vi "Read File interpreter.lvclass.vi"(8 "error in (no error)":errorcluster, 11 "AutoExp in":refnum<class "AutoExp.lvclass">) -> (0 "error out":errorcluster, 2 "File interpreter.lvclass":refnum<class "File interpreter.lvclass">, 3 "AutoExp out":refnum<class "AutoExp.lvclass">)   [LabVIEW 2018]
uses:
  AutoExp.lvclass
  File interpreter/File interpreter.lvclass
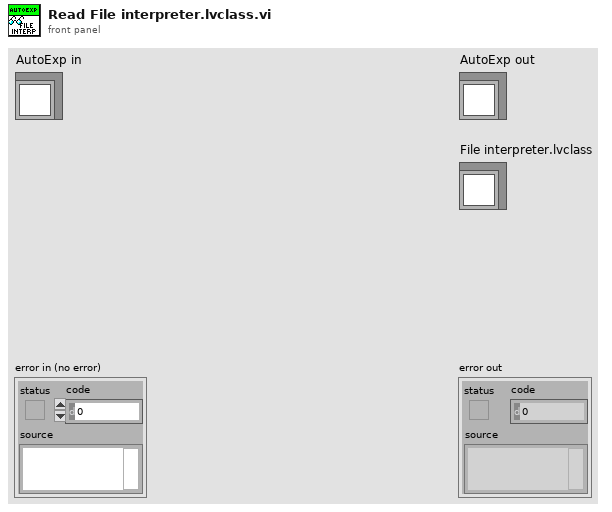
[diagram p1: front panel]
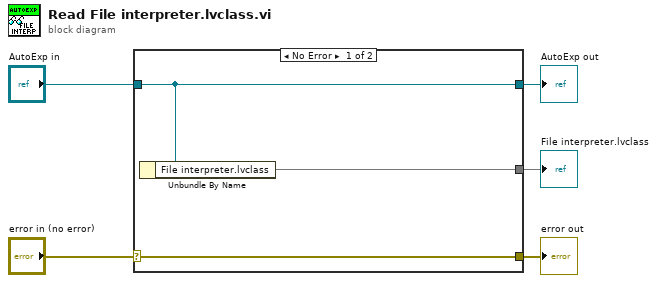
[diagram p0: block diagram]
diagram:
  n1 = case shown="No Error" "error in (no error)" {
    selector: "error in (no error)" -> [w8 w9]
    tunnel: [w8 w9] -> w4
    tunnel: [w7 w10] -> w2
    tunnel: "AutoExp in" -> [w7 w10]
    tunnel: [w6 _] -> w1
    frame No Error {
      n2 = Unbundle By Name(w7) -> ("File interpreter.lvclass"=w6)
    }
    frame Error {
    }
  }
  "error out" <- w4
  "AutoExp out" <- w2
  "File interpreter.lvclass" <- w1
